vi "fileUpTempWithSN&Date.vi"(0 "input_array_temp_int":u8[][](array[numeric]) format="%.0x", 1 "input_str_Date":string, 2 "input_str_SN":string, 3 "校验信息":T1(array[cluster]), 4 "input_str_customer":string, 7 "DateCode8Value_0X30":i32) -> (5 "show_array_temp_int":u8[][](array[numeric])=[[3, 4, 33, 0, 0, 0, 0, 65, 4, 128, 213, 0, 103, 0, 0, 0, 0, 0, 0, 0, 0, 0, 0, 0, 0, 0, 0, 0, 0, 0, 0, 0, 0, 0, 0, 0, 0, 0, 0, 0, 0, 0, 0, 0, 0, 0, 0, 0, 0, 0, 0, 0, 0, 0, 0, 0, 0, 0, 0, 0, 1, 0, 0, 42, 0, 0, 0, 0, 0, 0, 0, 0, 0, 0, 0, 0, 0, 0, 0, 0, 0, 0, 0, 0, 49, 52, 49, 49, 50, 53, 0, 0, 0, 0, 0, 46, 0, 0, 0, 0, 0, 0, 0, 0, 0, 0, 0, 0, 0, 0, 0, 0, 0, 0, 0, 0, 0, 0, 0, 0, 0, 0, 0, 0, 0, 0, 0, 0, 0, 0, 0, 0, 0, 0, 0, 0, 0, 0, 0, 0, 0, 0, 0, 0, 0, 0, 0, 0, 0, 0, 0, 0, 0, 0, 0, 0, 0, 0, 0, 0, 0, 0, 0, 0, 0, 0, 0, 0, 0, 0, 0, 0, 0, 0, 0, 0, 0, 0, 0, 0, 0, 0, 0, 0, 0, 0, 0, 0, 0, 0, 0, 0, 0, 0, 0, 0, 0, 0, 0, 0, 0, 0, 0, 0, 0, 0, 0, 0, 0, 0, 0, 0, 0, 0, 0, 0, 0, 0, 0, 0, 0, 0, 0, 0, 0, 0, 0, 0, 0, 0, 0, 0, 0, 0, 0, 0, 0, 0, 0, 0, 0, 0, 0, 0, 0, 0, 0, 0, 0, 0, 0, 0, 0, 0, 0, 0]] format="%.0x", 6 "Output String":string[](array[string]))   [LabVIEW 2011]
panel:
  # "file up template with SN and Date"
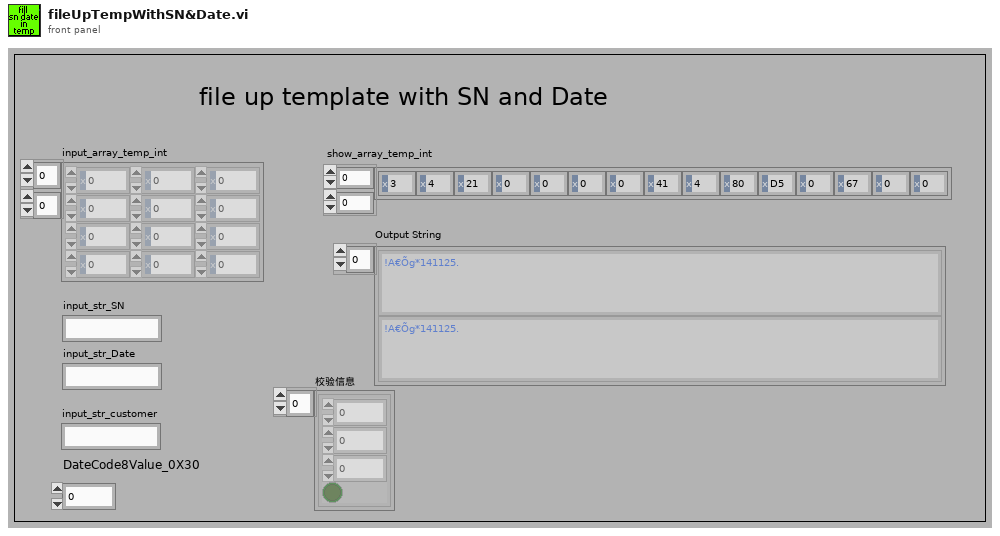
[diagram p1: front panel]
types:
  T1 = cluster{"start":i32, "length":i32, "p":i32, "H/L":bool}[]
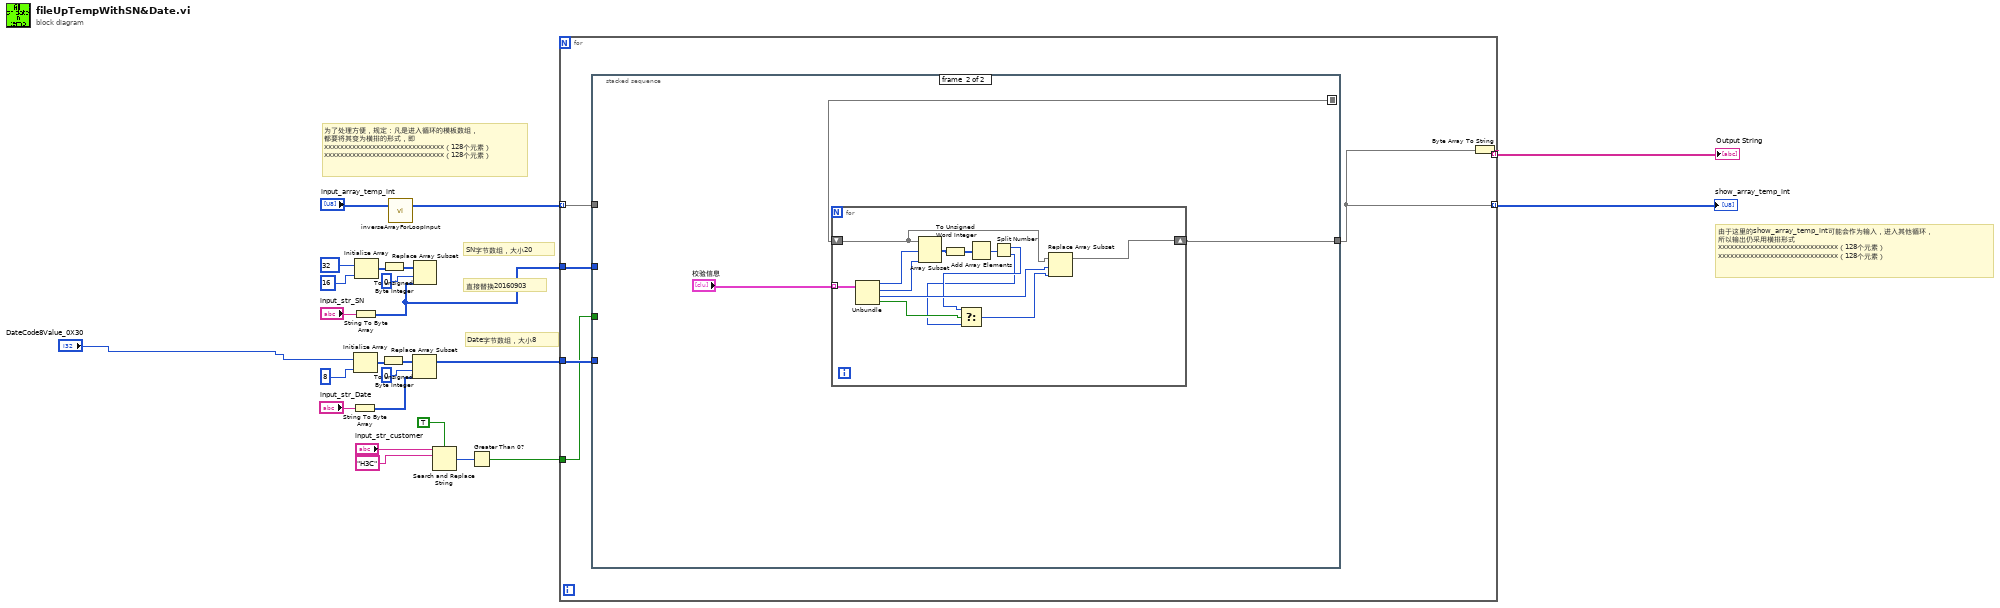
[diagram p0: block diagram]
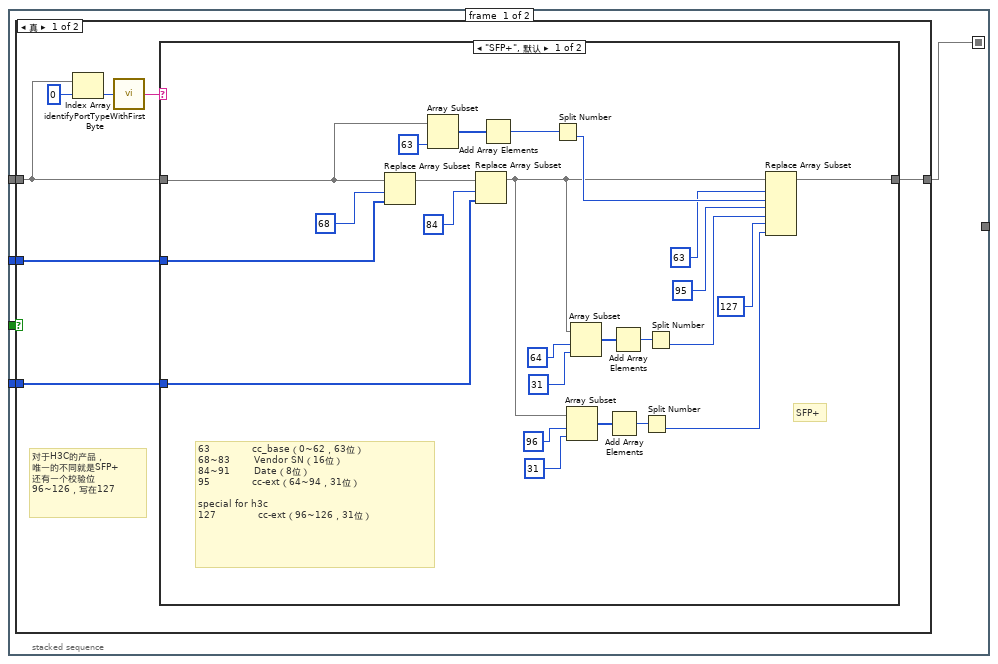
[diagram p2: hidden frame]
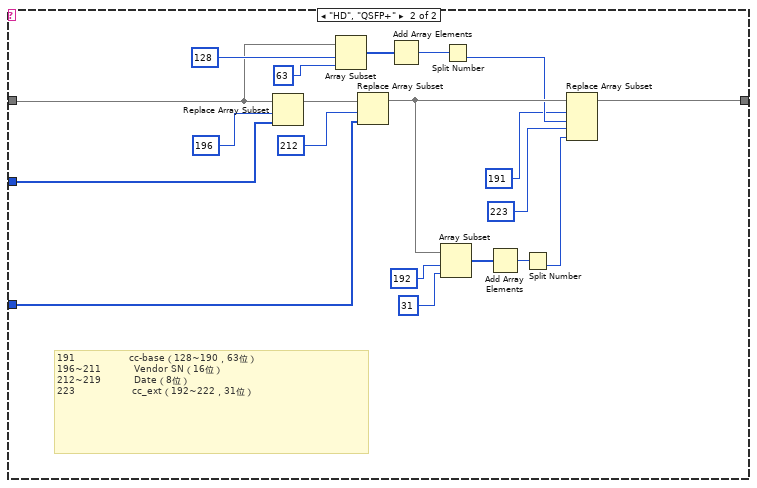
[diagram p3: hidden frame]
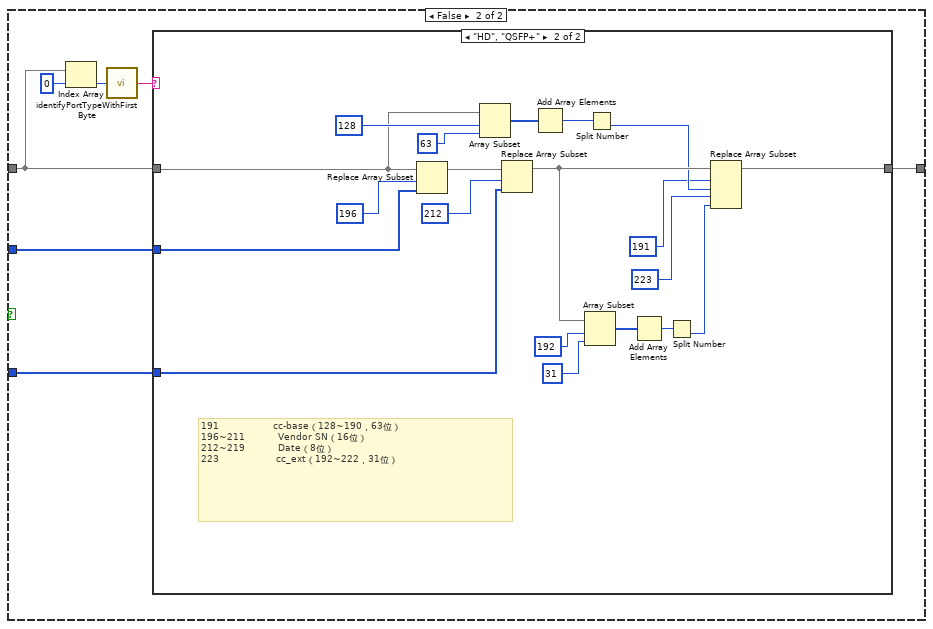
[diagram p4: hidden frame]
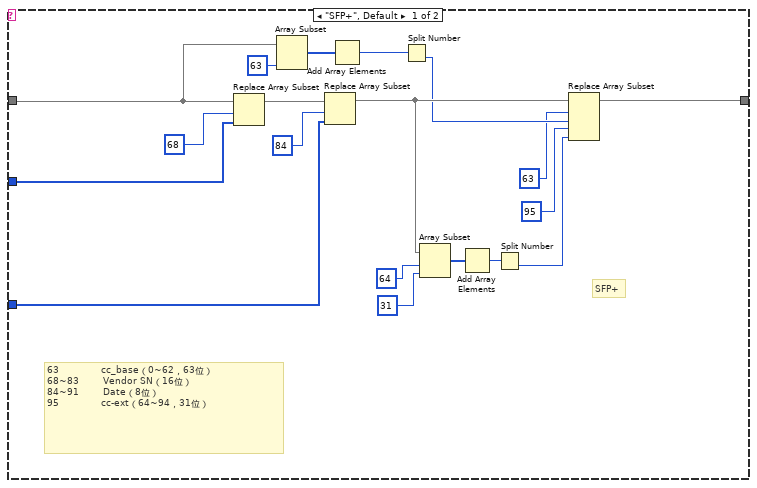
[diagram p5: hidden frame]
diagram:
  # "直接替换20160903"
  # "由于这里的show_array_temp_int可能会作为输入，进入其他循环，\n所以输出仍采用横排形式\nxxxxxxxxxxxxxxxxxxxxxxxxxxxxxx（128个元素）\nxxxxxxxxxxxxxxxxxxxxxxxxxxxxxx（128个元素）"
  # "Date字节数组，大小8"
  # "SN字节数组，大小20"
  # "为了处理方便，规定：凡是进入循环的模板数组，\n都要将其变为横排的形式，即\nxxxxxxxxxxxxxxxxxxxxxxxxxxxxxx（128个元素）\nxxxxxxxxxxxxxxxxxxxxxxxxxxxxxx（128个元素）"
  n1 = String To Byte Array(string="input_str_Date") -> (unsigned byte array=w15:u8[])
  n2 = String To Byte Array(string="input_str_SN") -> (unsigned byte array=w1:u8[])
  n3 = Initialize Array("DateCode8Value_0X30", 8 ("维数大小")) -> (w13:i32[])
  n4 = Initialize Array(32, 16 ("维数大小")) -> (w19:i32[])
  n5 = To Unsigned Byte Integer(number=w13) -> (unsigned 8bit integer=w14:u8[])
  n6 = To Unsigned Byte Integer(number=w19) -> (unsigned 8bit integer=w18:u8[])
  n7 = call "inverseArrayForLoopInput.vi"("input_array_temp_int"="input_array_temp_int") -> ("show_array_temp_int"=w23:u8[][])  [unwired: 1 in, 1 out]
  n8 = Replace Array Subset(array=w14, new element=w15, index=0 ("索引")) -> (w10:u8[])
  n9 = Replace Array Subset(array=w18, new element=w1, index=0 ("索引")) -> ()  [unwired: 1 out]
  n10 = Search and Replace String(case sensitive?=TRUE ("忽略大小写？(F)"), input string="input_str_customer", search string="H3C" ("搜索字符串")) -> (number of replacements=w4:i32)  [unwired: 5 in, 3 out]
  n11 = Greater Than 0?(x=w4) -> (x > 0?=w3:bool)
  n12 = for {
    tunnel: w23 -> [w30] mode=indexing
    tunnel: w1 -> [w29]
    tunnel: w10 -> [w28]
    tunnel: [w25] -> w9 mode=indexing
    tunnel: [w27] -> w8 mode=indexing
    tunnel: w3 -> [w26]
    n13 = stacked-sequence {
      seq-local: [w31 _] -> [_ w135]
      tunnel: w30 -> [w35 _]
      tunnel: w29 -> [w34 _]
      tunnel: w28 -> [w33 _]
      tunnel: w26 -> [w32 _]
      tunnel: [_ w134] -> w25
      frame #0 {
        n14 = case shown="真" w32 {
          tunnel: w35 -> [w39 w91]
          tunnel: w34 -> [w38 w90]
          tunnel: w33 -> [w37 w89]
          tunnel: [w36 w88] -> w31
          frame True {
            # "对于H3C的产品，\n唯一的不同就是SFP+\n还有一个校验位\n96~126，写在127"
            n15 = Index Array(array=w39, index=0 ("索引")) -> (element=w41:u8)
            n16 = call "identifyPortTypeWithFirstByte.vi"("input_int"=w41) -> ("show_str_portType"=w40:string)
            n17 = case shown="\"SFP+\", 默认" w40 {
              tunnel: w39 -> [w53 w71]
              tunnel: w38 -> [w52 w70]
              tunnel: w37 -> [w51 w69]
              tunnel: [w50 w68] -> w36
              frame "SFP+", Default {
                # "63              cc_base（0~62，63位）\n68~83        Vendor SN（16位）\n84~91        Date（8位）\n95              cc-ext（64~94，31位）\n\nspecial for h3c\n127              cc-ext（96~126，31位）"
                # "SFP+"
                n18 = Replace Array Subset(array=w53, new element=w52, index=68 ("索引")) -> (w61:u8[])
                n19 = Array Subset(array=w53, length=63 ("长度")) -> (w60:u8[])  [unwired: 1 in]
                n20 = Replace Array Subset(array=w61, new element=w51, index=84 ("索引")) -> (w45:u8[])
                n21 = Add Array Elements(numeric array=w60) -> (sum=w59:u8)
                n22 = Split Number(x=w59) -> (lo(x)=w62:u8)  [unwired: 1 out]
                n23 = Array Subset(array=w45, index=96 ("索引"), length=31 ("长度")) -> (w48:u8[])
                n24 = Array Subset(array=w45, index=64 ("索引"), length=31 ("长度")) -> (w64:u8[])
                n25 = Add Array Elements(numeric array=w48) -> (sum=w47:u8)
                n26 = Add Array Elements(numeric array=w64) -> (sum=w65:u8)
                n27 = Split Number(x=w47) -> (lo(x)=w44:u8)  [unwired: 1 out]
                n28 = Split Number(x=w65) -> (lo(x)=w67:u8)  [unwired: 1 out]
                n29 = Replace Array Subset(array=w45, new element #1=w62, index #1=63 ("索引"), new element #2=w67, index #2=95 ("索引"), new element #3=w44, index #3=127 ("索引")) -> (w50:u8[])
              }
              frame "HD", "QSFP+" {
                # "191                  cc-base（128~190，63位）\n196~211           Vendor SN（16位）\n212~219           Date（8位）\n223                   cc_ext（192~222，31位）"
                n30 = Replace Array Subset(array=w71, new element=w70, index=196 ("索引")) -> (w79:u8[])
                n31 = Array Subset(array=w71, index=128 ("长度"), length=63 ("长度")) -> (w78:u8[])
                n32 = Replace Array Subset(array=w79, new element=w69, index=212 ("索引")) -> (w85:u8[])
                n33 = Add Array Elements(numeric array=w78) -> (sum=w77:u8)
                n34 = Array Subset(array=w85, index=192 ("索引"), length=31 ("长度")) -> (w82:u8[])
                n35 = Split Number(x=w77) -> (lo(x)=w80:u8)  [unwired: 1 out]
                n36 = Add Array Elements(numeric array=w82) -> (sum=w83:u8)
                n37 = Split Number(x=w83) -> (lo(x)=w86:u8)  [unwired: 1 out]
                n38 = Replace Array Subset(array=w85, new element #1=w80, index #1=191 ("索引"), new element #2=w86, index #2=223 ("索引")) -> (w68:u8[])
              }
            }
          }
          frame False {
            n39 = Index Array(array=w91, index=0 ("索引")) -> (element=w93:u8)
            n40 = call "identifyPortTypeWithFirstByte.vi"("input_int"=w93) -> ("show_str_portType"=w92:string)
            n41 = case shown="\"HD\", \"QSFP+\"" w92 {
              tunnel: w91 -> [w98 w117]
              tunnel: w90 -> [w97 w116]
              tunnel: w89 -> [w96 w115]
              tunnel: [w95 w114] -> w88
              frame "SFP+", Default {
                # "63              cc_base（0~62，63位）\n68~83        Vendor SN（16位）\n84~91        Date（8位）\n95              cc-ext（64~94，31位）"
                # "SFP+"
                n42 = Replace Array Subset(array=w98, new element=w97, index=68 ("索引")) -> (w106:u8[])
                n43 = Array Subset(array=w98, length=63 ("长度")) -> (w105:u8[])  [unwired: 1 in]
                n44 = Replace Array Subset(array=w106, new element=w96, index=84 ("索引")) -> (w112:u8[])
                n45 = Add Array Elements(numeric array=w105) -> (sum=w104:u8)
                n46 = Split Number(x=w104) -> (lo(x)=w107:u8)  [unwired: 1 out]
                n47 = Array Subset(array=w112, index=64 ("索引"), length=31 ("长度")) -> (w109:u8[])
                n48 = Add Array Elements(numeric array=w109) -> (sum=w110:u8)
                n49 = Split Number(x=w110) -> (lo(x)=w113:u8)  [unwired: 1 out]
                n50 = Replace Array Subset(array=w112, new element #1=w107, index #1=63 ("索引"), new element #2=w113, index #2=95 ("索引")) -> (w95:u8[])
              }
              frame "HD", "QSFP+" {
                # "191                  cc-base（128~190，63位）\n196~211           Vendor SN（16位）\n212~219           Date（8位）\n223                   cc_ext（192~222，31位）"
                n51 = Replace Array Subset(array=w117, new element=w116, index=196 ("索引")) -> (w125:u8[])
                n52 = Array Subset(array=w117, index=128 ("长度"), length=63 ("长度")) -> (w124:u8[])
                n53 = Replace Array Subset(array=w125, new element=w115, index=212 ("索引")) -> (w131:u8[])
                n54 = Add Array Elements(numeric array=w124) -> (sum=w123:u8)
                n55 = Array Subset(array=w131, index=192 ("索引"), length=31 ("长度")) -> (w128:u8[])
                n56 = Split Number(x=w123) -> (lo(x)=w126:u8)  [unwired: 1 out]
                n57 = Add Array Elements(numeric array=w128) -> (sum=w129:u8)
                n58 = Split Number(x=w129) -> (lo(x)=w132:u8)  [unwired: 1 out]
                n59 = Replace Array Subset(array=w131, new element #1=w126, index #1=191 ("索引"), new element #2=w132, index #2=223 ("索引")) -> (w114:u8[])
              }
            }
          }
        }
      }
      frame #1 {
        n60 = for {
          tunnel: "校验信息" -> [w149] mode=indexing
          shift-right: [w139] -> w134
          shift-left: w135 -> [w145]
          n61 = Unbundle(w149) -> ("start"=w147:i32, "length"=w146:i32, "p"=w144:i32, "H/L"=w143:bool)
          n62 = Array Subset(array=w145, index=w147, length=w146) -> (w138:u8[])
          n63 = To Unsigned Word Integer(number=w138) -> (unsigned 16bit integer=w137:u16[])
          n64 = Add Array Elements(numeric array=w137) -> (sum=w148:u16)
          n65 = Split Number(x=w148) -> (hi(x)=w142:u8, lo(x)=w141:u8)
          n66 = Select(t=w142, s=w143, f=w141) -> (s? t:f=w140:u8)
          n67 = Replace Array Subset(array=w145, new element=w140, index=w144) -> (w139:u8[])
        }
      }
    }
    n68 = Byte Array To String(unsigned byte array=w25) -> (string=w27:string)
  }
  "show_array_temp_int" <- w9
  "Output String" <- w8
